vi "Calc_Msg_Type.vi"(0 "Element Values":enum8{"False", "True", "Mixed"}[](array[ring])) -> (1 "BuildType":T1=6 items=["simple", "Dialog", "PVUpdate", "Dialog&PV", "Asynch", "AsynchDial", "Ack"], 2 "Symbol Index":i32=7)   [LabVIEW 2016, in "CS++MessageMakerMain.lvlib" / "CS++MessageMakerMain.lvclass"]
uses:
  CS++MessageMakerMain.lvclass
  BuildType.ctl
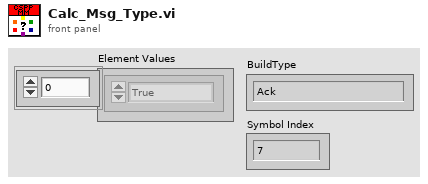
[diagram p1: front panel]
types:
  T1 = typedef "CS++MessageMakerMain.lvlib/CS++MessageMakerMain.lvclass/BuildType.ctl" = u16
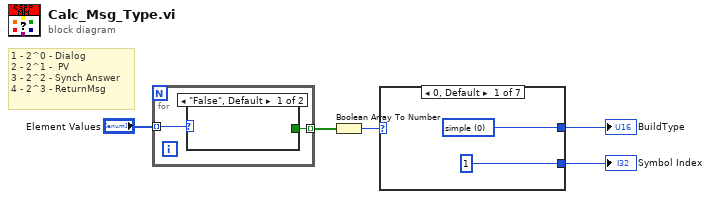
[diagram p0: block diagram]
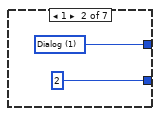
[diagram p2: hidden frame]
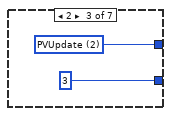
[diagram p3: hidden frame]
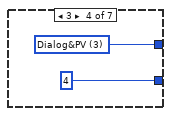
[diagram p4: hidden frame]
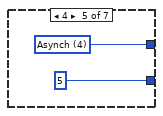
[diagram p5: hidden frame]
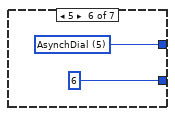
[diagram p6: hidden frame]
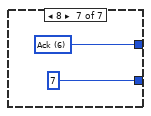
[diagram p7: hidden frame]
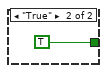
[diagram p8: hidden frame]
diagram:
  # "1 - 2^0 - Dialog\n2 - 2^1 -  PV\n3 - 2^2 - Synch Answer\n4 - 2^3 - ReturnMsg"
  n1 = for {
    tunnel: "Element Values" -> [w7] mode=indexing
    tunnel: [w6] -> w4 mode=indexing
    n2 = case shown="\"False\", Default" w7 {
      tunnel: [_ TRUE] -> w6
      frame "False", Default {
      }
      frame "True" {
      }
    }
  }
  n3 = Boolean Array To Number(Boolean array=w4) -> (number=w3:u32)
  n4 = case shown="0, Default" w3 {
    tunnel: [w10 w12 w14 w16 w18 w20 w22] -> w2
    tunnel: [1 ("Active Item:Symbol Index") 2 ("Active Item:Symbol Index") 3 ("Active Item:Symbol Index") 4 ("Active Item:Symbol Index") 5 ("Active Item:Symbol Index") 6 ("Active Item:Symbol Index") 7 ("Active Item:Symbol Index")] -> w1
    frame 0, Default {
      w10 = T1 0 items=["simple", "Dialog", "PVUpdate", "Dialog&PV", "Asynch", "AsynchDial", "Ack"] ("BuildType")
    }
    frame 1 {
      w12 = T1 1 items=["simple", "Dialog", "PVUpdate", "Dialog&PV", "Asynch", "AsynchDial", "Ack"] ("BuildType")
    }
    frame 2 {
      w14 = T1 2 items=["simple", "Dialog", "PVUpdate", "Dialog&PV", "Asynch", "AsynchDial", "Ack"] ("BuildType")
    }
    frame 3 {
      w16 = T1 3 items=["simple", "Dialog", "PVUpdate", "Dialog&PV", "Asynch", "AsynchDial", "Ack"] ("BuildType")
    }
    frame 4 {
      w18 = T1 4 items=["simple", "Dialog", "PVUpdate", "Dialog&PV", "Asynch", "AsynchDial", "Ack"] ("BuildType")
    }
    frame 5 {
      w20 = T1 5 items=["simple", "Dialog", "PVUpdate", "Dialog&PV", "Asynch", "AsynchDial", "Ack"] ("BuildType")
    }
    frame 8 {
      w22 = T1 6 items=["simple", "Dialog", "PVUpdate", "Dialog&PV", "Asynch", "AsynchDial", "Ack"] ("BuildType")
    }
  }
  "BuildType" <- w2
  "Symbol Index" <- w1
